vi "Initialize FPGA Board.vi"(8 "error in":errorcluster, 10 "Redetect?":bool, 11 "FPGA VI Reference In":refnum<k20>) -> (0 "error out":errorcluster, 3 "FPGA VI Reference Out":refnum<k20>)   [LabVIEW 2012]
doc: "This VI initializes adpater mddule"
uses:
  <vilib>/FPGAPlugInAG/Dynamic/niLvFpga_Reset_Dynamic.vi
  <vilib>/LabVIEW Targets/FPGA/FlexRIO/CustomFPGAMethods/79XXR_Method_RedetectIOModuleImpl.vi
  <vilib>/FPGAPlugInAG/Dynamic/niLvFpga_Run_Dynamic.vi
  <vilib>/rvi/interface/nirviMethod/nirviMethod.xnode
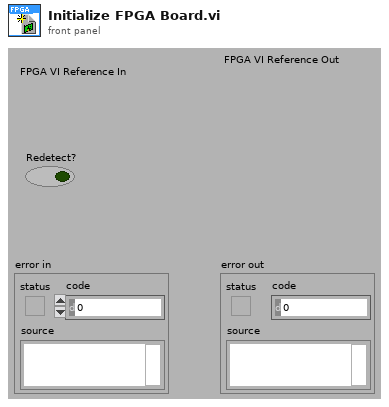
[diagram p1: front panel]
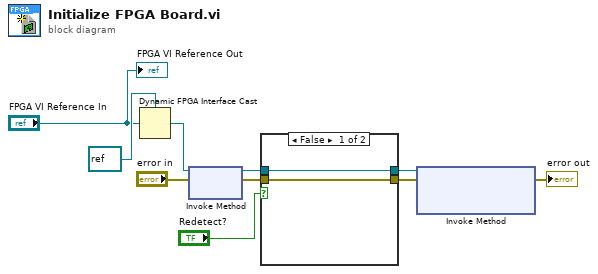
[diagram p0: block diagram]
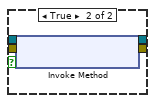
[diagram p2: hidden frame]
diagram:
  n1 = Dynamic FPGA Interface Cast(Session In=refnum<k20> refnum ("Type"), Type="FPGA VI Reference In") -> (Session Out=w7:refnum<k20>)
  n2 = xnode "Invoke Method"("FPGA VI Reference In"=w7, "error in"="error in") -> ("FPGA VI Reference Out"=w6:refnum<k20>, "error out"=w5:errorcluster)
  n3 = case shown="False" "Redetect?" {
    tunnel: w6 -> [w12 w16]
    tunnel: w5 -> [w11 w15]
    tunnel: [w11 w14] -> w4
    tunnel: [w12 w13] -> w3
    frame False {
    }
    frame True {
      n4 = xnode "Invoke Method"("FPGA VI Reference In"=w16, "error in"=w15) -> ("FPGA VI Reference Out"=w13:refnum<k20>, "error out"=w14:errorcluster)
    }
  }
  n5 = xnode "Invoke Method"("FPGA VI Reference In"=w3, "error in"=w4) -> ("error out"=→"error out":errorcluster)  [unwired: 1 in, 1 out]
  "FPGA VI Reference Out" <- "FPGA VI Reference In"
